vi "Weather Station Sandbox.vi"() -> ()   [LabVIEW 2011]
uses:
  Classes/IP Connection/IP Connection.lvclass
  Classes/Ambient Light Bricklet/Ambient Light Bricklet.lvclass
  Classes/Humidity Bricklet/Humidity Bricklet.lvclass
  Classes/Temperature IR Bricklet/Temperature IR Bricklet.lvclass
  Classes/Barometer Bricklet/Barometer Bricklet.lvclass
panel:
  out "Air Pressure":dbl format="%.3f mbar"
  out "Illuminance":dbl format="%.1f Lux"
  out "Humidity":dbl format="%.1f %%"
  out "Object T.":dbl format="%.1f °C"
  out "Ambient T.":dbl format="%.1f °C"
  out "XY Graph":cluster{dbl[], dbl[]}[](graph)
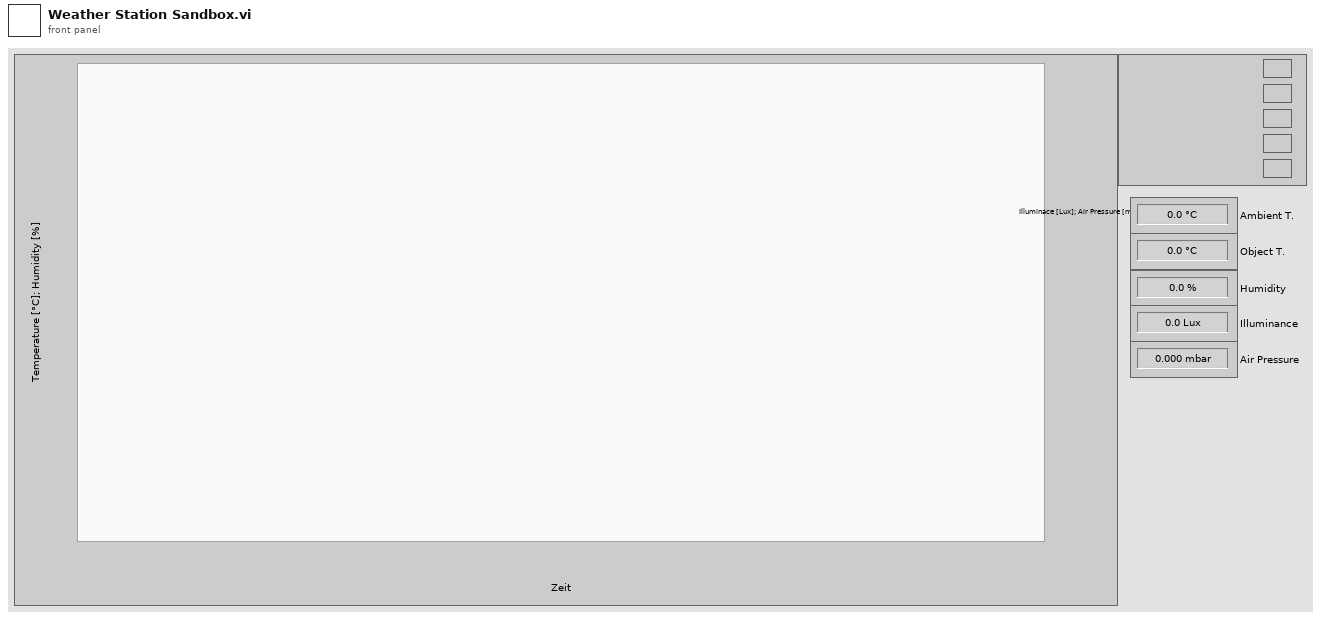
[diagram p1: front panel]
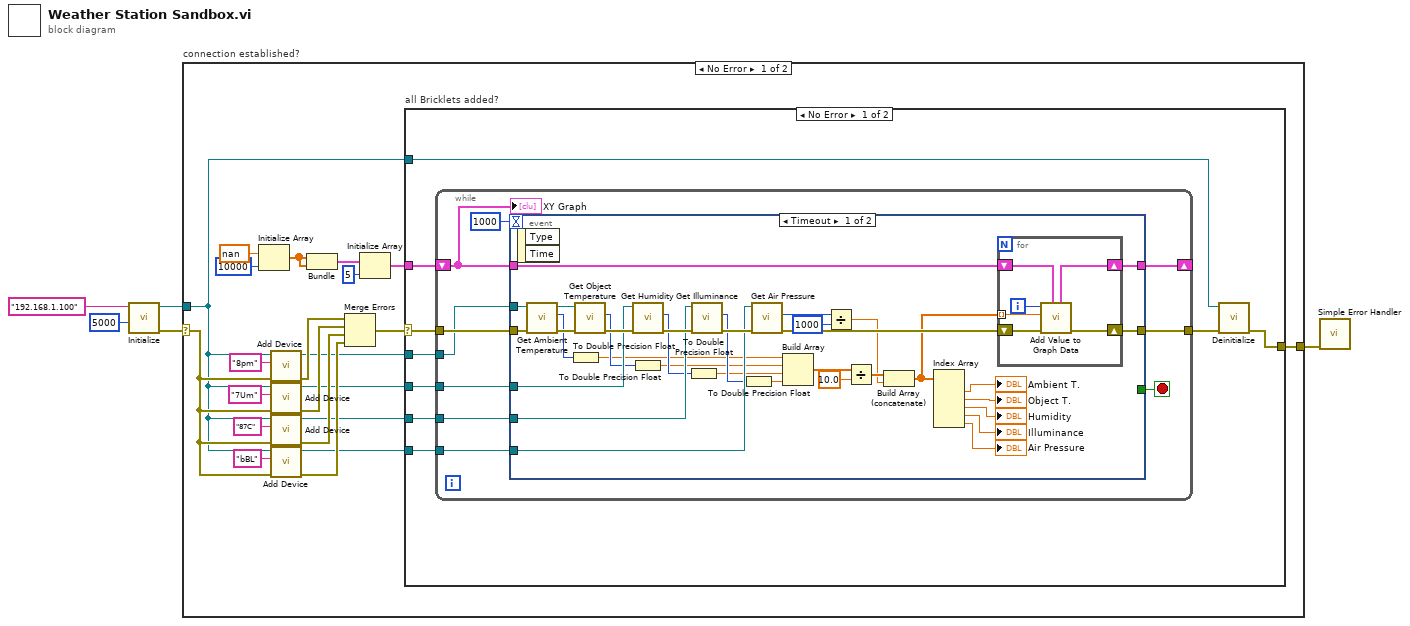
[diagram p0: block diagram]
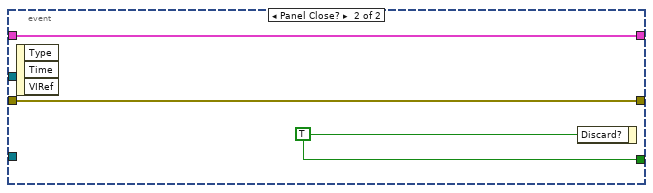
[diagram p2: hidden frame]
diagram:
  n1 = call "Initialize.vi"("Timeout (2500ms)"=5000, "IP (localhost)"="192.168.1.100") -> ("error out"=w5:errorcluster, "IP Connection out"=w4:refnum<class "IP Connection.lvclass">)  [unwired: 8 in]
  n2 = case "connection established?" shown="No Error" w5 {
    selector: w5 -> [w22 w91]
    tunnel: w4 -> [w21 _]
    tunnel: [w24 w91] -> w3
    frame No Error {
      n3 = Initialize Array(nan ("element"), 10000 ("dimension size")) -> (w13:dbl[])
      n4 = call "Add Device.vi"("Error In"=w22, "Device UID"="8pm", "IP Connection"=w21) -> ("Error Out"=w19:errorcluster, "Ambient Light Bricklet"=w9:refnum<class "Temperature IR Bricklet.lvclass">)  [unwired: 7 in]
      n5 = call "Add Device.vi"("Error In"=w22, "Device UID"="7Um", "IP Connection"=w21) -> ("Error Out"=w18:errorcluster, "Humidity Bricklet"=w8:refnum<class "Humidity Bricklet.lvclass">)  [unwired: 7 in]
      n6 = call "Add Device.vi"("Error In"=w22, "Device UID"="87C", "IP Connection"=w21) -> ("Error Out"=w17:errorcluster, "Ambient Light Bricklet"=w7:refnum<class "Ambient Light Bricklet.lvclass">)  [unwired: 7 in]
      n7 = call "Add Device.vi"("Error In"=w22, "Device UID"="bBL", "IP Connection"=w21) -> ("Error Out"=w16:errorcluster, "Barometer Bricklet"=w6:refnum<class "Barometer Bricklet.lvclass">)  [unwired: 7 in]
      n8 = Bundle(w13, w13) -> (w14:cluster{dbl[], dbl[]})  [unwired: 1 in]
      n9 = Merge Errors(w19, w18, w17, w16) -> (w23:errorcluster)
      n10 = Initialize Array(w14, 5 ("dimension size")) -> (w10:cluster{dbl[], dbl[]}[])
      n11 = case "all Bricklets added?" shown="No Error" w23 {
        selector: w23 -> [w32 w90]
        tunnel: [w34 w90] -> w24
        tunnel: w21 -> [w35 _]
        tunnel: w10 -> [w33 _]
        tunnel: w9 -> [w31 _]
        tunnel: w8 -> [w30 _]
        tunnel: w7 -> [w29 _]
        tunnel: w6 -> [w28 _]
        frame No Error {
          n12 = while {
            tunnel: [w46] -> w36
            shift-right: [w43] -> _
            shift-left: w33 -> [w44]
            tunnel: w32 -> [w41]
            tunnel: w31 -> [w37]
            tunnel: w30 -> [w40]
            tunnel: w29 -> [w39]
            tunnel: w28 -> [w38]
            stop <- w45 stop-if-true
            n13 = event shown="[0] Timeout" {
              selector: _ -> [_ _]
              dyn-events: _ -> [_ _]
              timeout: 1000 -> [_ _]
              tunnel: [w68 w87] -> w46
              tunnel: [_ w89] -> w45
              tunnel: w44 -> [w69 w88]
              tunnel: [w67 w88] -> w43
              tunnel: w41 -> [w80 w87]
              tunnel: w40 -> [w73 _]
              tunnel: w39 -> [w72 _]
              tunnel: w38 -> [w71 _]
              tunnel: w37 -> [w79 _]
              event Timeout {
                n14 = event-data() -> ()  [unwired: 1 in, 2 out]
                n15 = call "Get Ambient Temperature.vi"("error in (no error)"=w80, "Temperature IR Bricklet in"=w79) -> ("error out"=w78:errorcluster, "Ambient Temperature"=w66:i16, "Temperature IR Bricklet out"=w77:refnum<class "Temperature IR Bricklet.lvclass">)  [unwired: 7 in]
                n16 = To Double Precision Float(number=w66) -> (double precision float=w62:dbl)
                n17 = call "Get Object Temperature.vi"("error in (no error)"=w78, "Temperature IR Bricklet in"=w77) -> ("error out"=w76:errorcluster, "Object Temperature"=w65:i16)  [unwired: 7 in, 1 out]
                n18 = call "Get Humidity.vi"("error in (no error)"=w76, "Humidity Bricklet in"=w73) -> ("error out"=w75:errorcluster, "Humidity"=w64:u16)  [unwired: 7 in, 1 out]
                n19 = To Double Precision Float(number=w65) -> (double precision float=w61:dbl)
                n20 = To Double Precision Float(number=w64) -> (double precision float=w60:dbl)
                n21 = call "Get Illuminance.vi"("error in (no error)"=w75, "Ambient Light Bricklet in"=w72) -> ("error out"=w74:errorcluster, "Illuminance"=w63:u16)  [unwired: 7 in, 1 out]
                n22 = To Double Precision Float(number=w63) -> (double precision float=w59:dbl)
                n23 = call "Get Air Pressure.vi"("error in (no error)"=w74, "Barometer Bricklet in"=w71) -> ("error out"=w70:errorcluster, "Air Pressure"=w56:i32)  [unwired: 7 in, 1 out]
                n24 = Build Array(w62, w61, w60, w59) -> (w58:dbl[])
                n25 = Divide(x=w56, y=1000) -> (x/y=w53:dbl)
                n26 = Divide(x=w58, y=10.0) -> (x/y=w54:dbl[])
                n27 = Build Array (concatenate)(w54, w53) -> (w52:dbl[])
                n28 = Index Array(array=w52) -> (element #1=→"Ambient T.":dbl, element #2=→"Object T.":dbl, element #3=→"Humidity":dbl, element #4=→"Illuminance":dbl, element #5=→"Air Pressure":dbl)  [unwired: 5 in]
                n29 = for {
                  shift-right: [w85] -> w68
                  shift-left: w70 -> [w86]
                  shift-right: [w84] -> w67
                  shift-left: w69 -> [w83]
                  tunnel: w52 -> [w81] mode=indexing
                  i -> [w82]
                  n30 = call "Add Value to Graph Data.vi"("Graph Data in"=w83, "Error In"=w86, "Value"=w81, "Index"=w82) -> ("Error Out"=w85:errorcluster, "Graph Data out"=w84:cluster{"Array":dbl[], "Array":dbl[]}[])  [unwired: 6 in]
                }
              }
              event Panel Close? {
                w89 = TRUE ("Discard?")
                n31 = event-data() -> ()  [unwired: 1 in, 3 out]
                n32 = event-data("Discard?"=w89) -> ()  [unwired: 1 in, 1 out]
              }
            }
            "XY Graph" <- w44
          }
          n33 = call "Deinitialize.vi"("error in (no error)"=w36, "IP Connection in"=w35) -> ("error out"=w34:errorcluster)  [unwired: 9 in]
        }
        frame Error {
        }
      }
    }
    frame Error {
    }
  }
  n34 = call <vilib>:"Simple Error Handler.vi"("error in (no error)"=w3) -> ()  [unwired: 4 in, 5 out]
